vi "fgv_vlp16_setting.vi"(7 "cmd":T3(ring), 8 "error in":errorcluster, 10 "VLP16 Mounting Offset in":T1 {"Z_Rotation[Deg]" format="%#.2f"; "Y_Rotation[Deg]" format="%#.2f"; "X_Rotation[Deg]" format="%#.2f"; "Z_offset[m]" format="%#.2f"; "Y_offset[m]" format="%#.2f"; "X_offset[m]" format="%#.2f"}, 11 "vlp-16 range setting in":T2={"x range"=20.0, "y range Max"=10.0, "y range Min"=-10.0, "z range"=1.0}) -> (0 "error out":errorcluster, 2 "VLP16 Mounting Offset out":T1, 3 "vlp-16 range setting out":T2={"x range"=20.0, "y range Max"=10.0, "y range Min"=-10.0, "z range"=1.0})   [LabVIEW 2019]
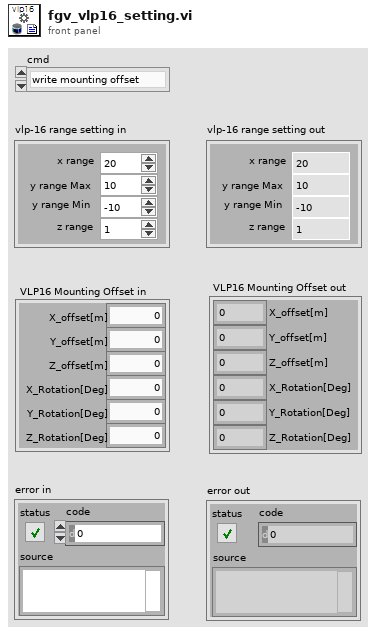
[diagram p1: front panel]
types:
  T1 = cluster{"X_offset[m]":sgl, "Y_offset[m]":sgl, "Z_offset[m]":sgl, "X_Rotation[Deg]":sgl, "Y_Rotation[Deg]":sgl, "Z_Rotation[Deg]":sgl}
  T2 = cluster{"x range":dbl, "y range Max":dbl, "y range Min":dbl, "z range":dbl}
  T3 = enum16{"write mounting offset", "write range setting", "read"}
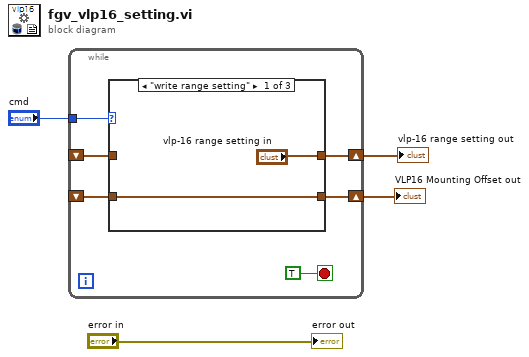
[diagram p0: block diagram]
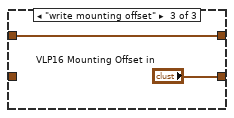
[diagram p3: hidden frame]
diagram:
  n1 = while {
    tunnel: "cmd" -> [w9]
    shift-right: [w8] -> w3
    shift-left: _ -> [w7]
    shift-right: [w6] -> w2
    shift-left: _ -> [w5]
    stop <- TRUE stop-if-true
    n2 = case shown="\"write range setting\"" w9 {
      tunnel: ["vlp-16 range setting in" w14 w16] -> w8
      tunnel: w7 -> [_ w14 w16]
      tunnel: [w11 w13 "VLP16 Mounting Offset in"] -> w6
      tunnel: w5 -> [w11 w13 _]
      frame "write range setting" {
      }
      frame "read", Default {
      }
      frame "write mounting offset" {
      }
    }
  }
  "vlp-16 range setting out" <- w3
  "VLP16 Mounting Offset out" <- w2
  "error out" <- "error in"
